vi "Main.vi"() -> ()   [LabVIEW 2014]
doc: "This Continuous Measurement sample project is based on the Queued Message Handler template.\n\nThe Event Handling Loop generates messages based on user interface actions.\n\nThe Message Handling Loop processes messages generated by the Event Handling Loop, or by other messages. There are also Acquisition and Logging message handling loop subVIs, and a chart updating loop."
uses:
  eod2016/controls/Recording Metadata.ctl
  Settings/Settings.ctl
  Acquisition/Hardware Configuration.ctl
  Logging/Logging Configuration.ctl
  controls/UI Data.ctl
  controls/UI State.ctl
  support/Message Queue/Enqueue Message (Single).vi
  <vilib>/Utility/error.llb/Error Cluster From Error Code.vi
  <vilib>/ErrorRing/Error Ring.xnode
  Acquisition/Acquisition.lvlib
  Logging/Logging.lvlib
  Settings/Settings.lvlib
  support/User Event - Stop/User Event - Stop.lvlib
  support/Message Queue/Message Queue.lvlib
panel:
  in  "UserMetaData":T1 {"Amplifier Model" items=["Select a Model", "AM 1700", "BMA 200"]}
  out "Data":waveform(dbl)[](graph)
  in  "Settings":bool
  in  "Start":bool
  in  "Stop":bool
  out "Status":string
  in  "Exit":bool
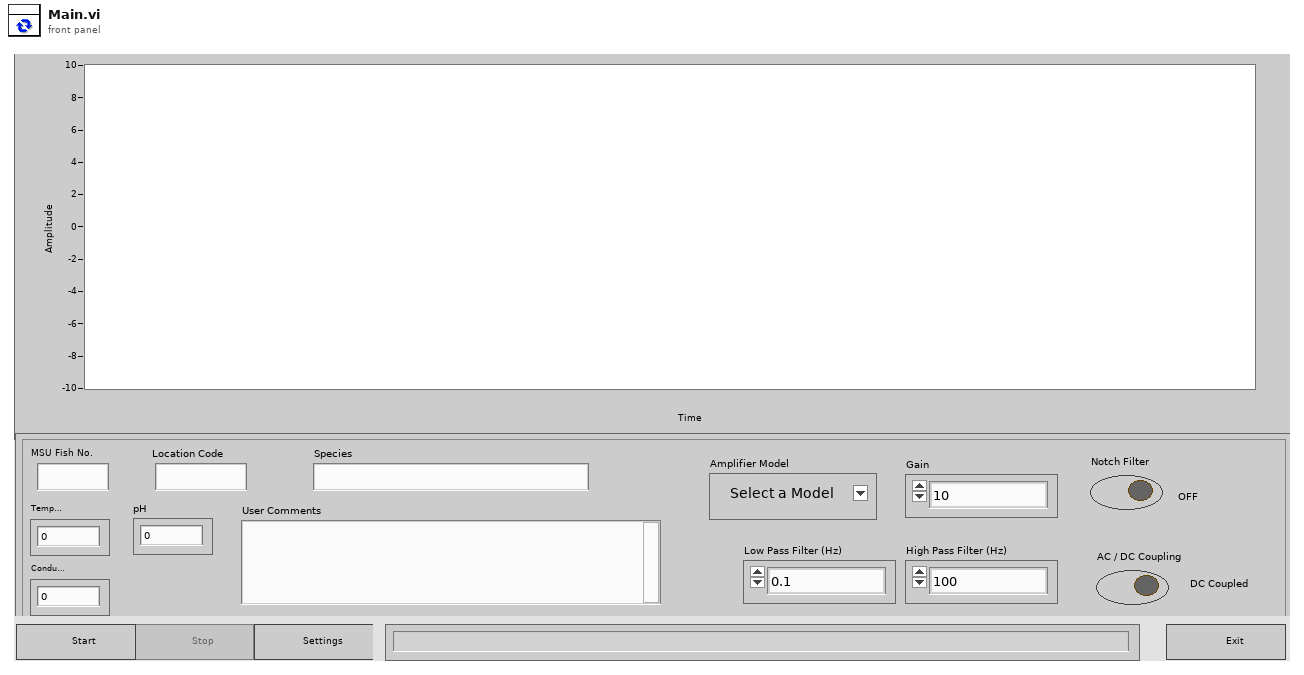
[diagram p1: front panel]
types:
  T1 = typedef "Recording Metadata.ctl" = cluster{"MSU Fish No.":string, "Location Code":string, "Species":string, "Temperature":dbl, "pH":dbl, "Conductivity":dbl, "User Comments":string, "Amplifier Model":u16, "Gain":enum16{"10", "20", "50", "100", "200", "500", "1000", "2k", "5k", "10k", "20k", "50k"}, "Low Pass Filter (Hz)":enum16{"0.1", "1", "3", "10", "30", "100", "300"}, "High Pass Filter (Hz)":enum16{"100", "500", "1000", "3000", "5000", "10,000", "20,000", "30,000", "50,000"}, "AC / DC Coupling":bool, "Notch Filter":bool}
  T2 = typedef "UI State.ctl" = enum16{"Idle", "Acquiring and Logging", "Waiting for Exit", "Waiting for Exit (Acq Stopped)", "Waiting for Exit (Log Stopped)", "Waiting for Stop", "Waiting for Stop (Acq Stopped)", "Waiting for Stop (Log Stopped)"}
  T3 = typedef "UI Data.ctl" = cluster{"Start Ref":refnum<vi>, "Trigger Ref":refnum<vi>, "Stop Ref":refnum<vi>, "Settings Ref":refnum<vi>, "Status Ref":refnum<vi>, "Exit Ref":refnum<vi>, "Data Ref":refnum<vi>}
  T4 = typedef "Settings.lvlib/Settings.ctl" = cluster{"Hardware Configuration":T5, "Logging Configuration":T6}
  T5 = typedef "Acquisition.lvlib/Hardware Configuration.ctl" = cluster{"DAQmx Channel":tag, "Max Input":dbl, "Min Input":dbl, "Sample Rate":dbl, "DAQmx Task":refnum<k21>}
  T6 = typedef "Logging.lvlib/Logging Configuration.ctl" = cluster{"Log File Base Path":path, "TDMS File Reference":refnum<k34>, "Samples to Save":u32, "InterRecording Delay":dbl}
  T7 = typedef "Message Queue.lvlib/All Message Queues.ctl" = cluster{"UI":refnum<queue>, "Acquisition":refnum<queue>, "Logging":refnum<queue>, "Timer":refnum<queue>}
  T8 = enum8{"Enabled", "Disabled", "Disabled and Grayed Out"}
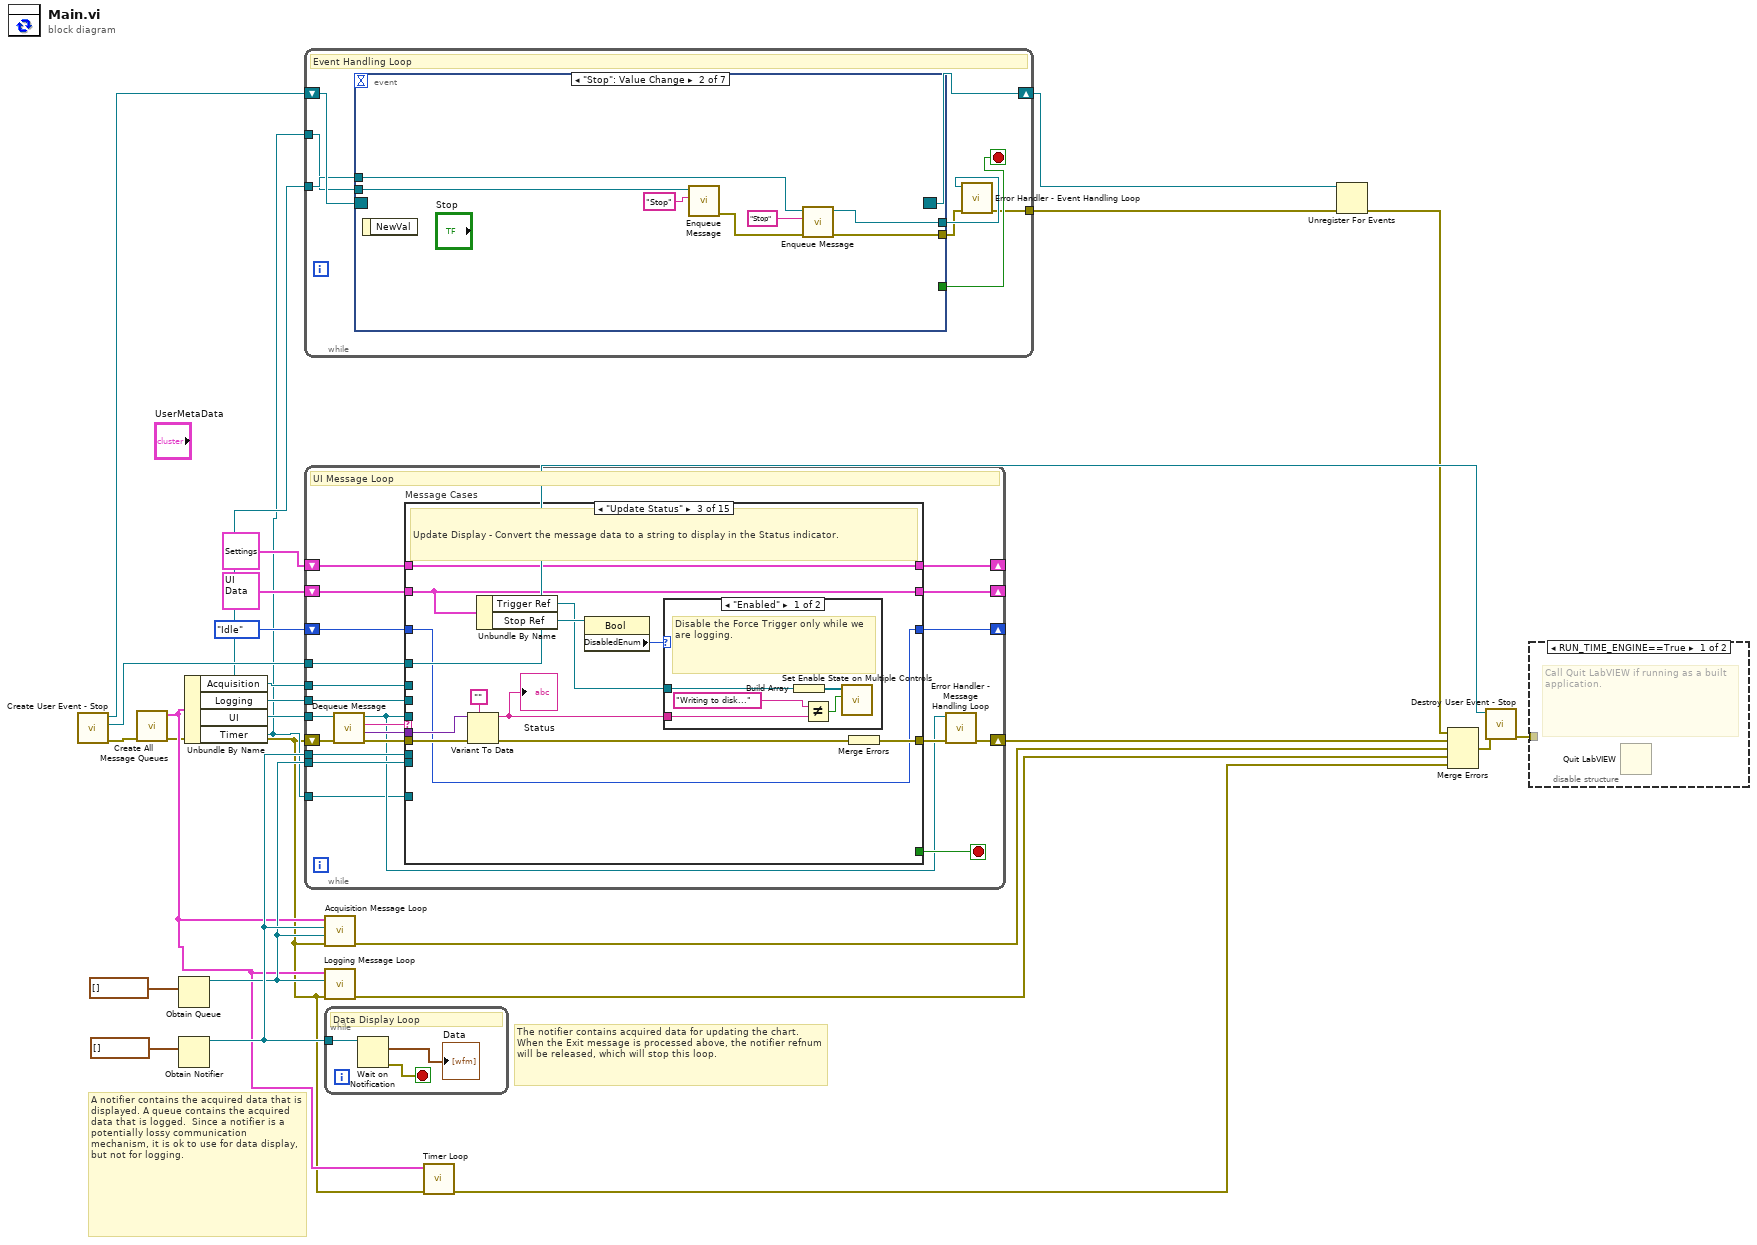
[diagram p0: block diagram]
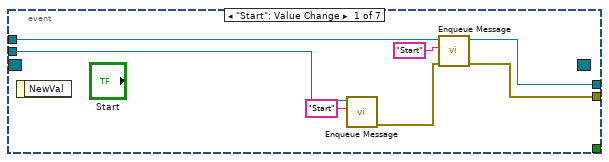
[diagram p3: hidden frame]
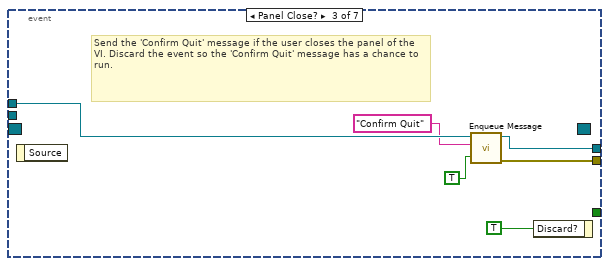
[diagram p4: hidden frame]
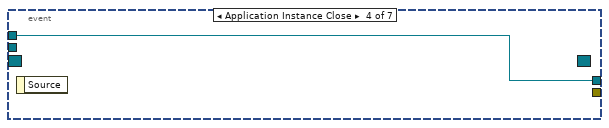
[diagram p5: hidden frame]
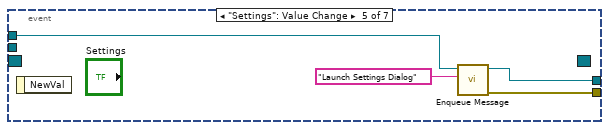
[diagram p6: hidden frame]
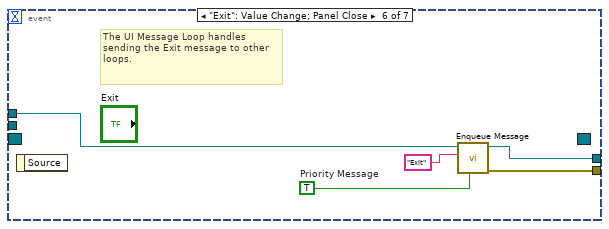
[diagram p7: hidden frame]
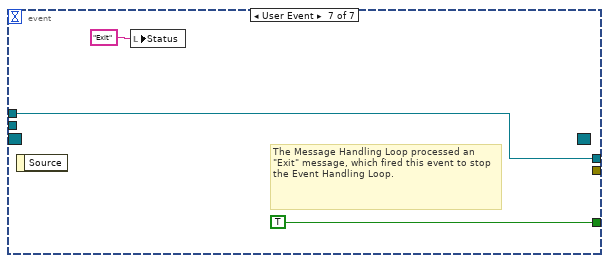
[diagram p8: hidden frame]
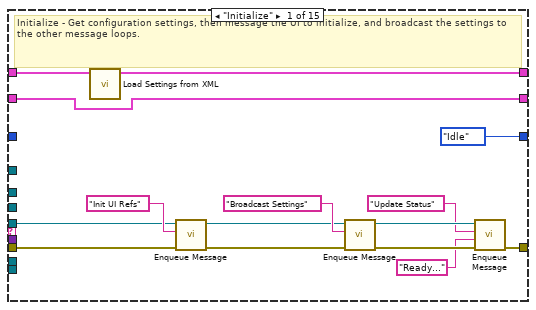
[diagram p9: hidden frame]
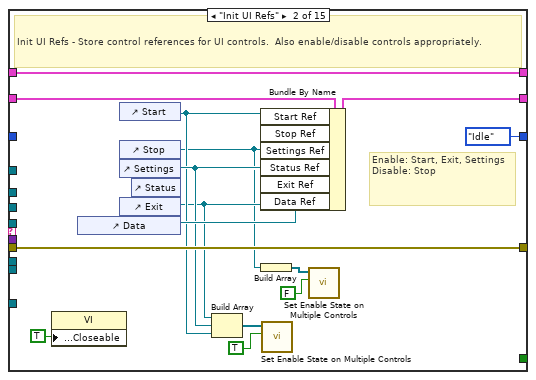
[diagram p10: hidden frame]
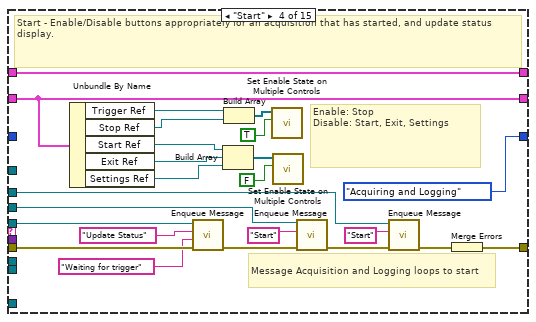
[diagram p12: hidden frame]
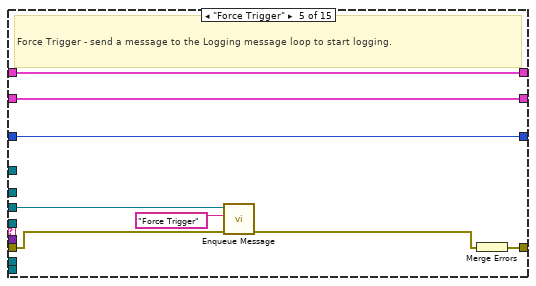
[diagram p13: hidden frame]
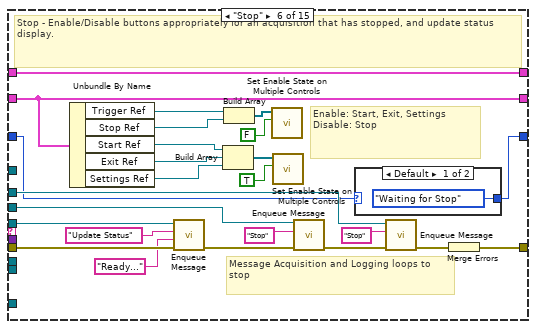
[diagram p14: hidden frame]
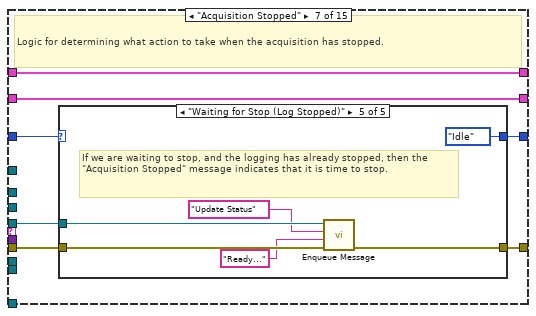
[diagram p16: hidden frame]
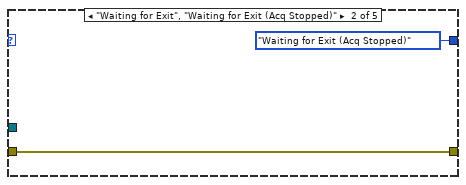
[diagram p18: hidden frame]
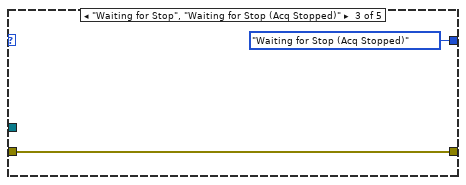
[diagram p19: hidden frame]
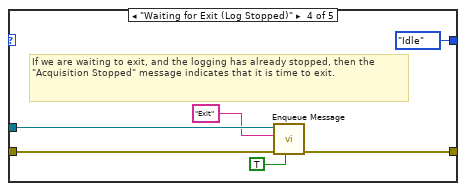
[diagram p20: hidden frame]
diagram:
  # "A notifier contains the acquired data that is displayed. A queue contains the acquired data that is logged.  Since a notifier is a potentially lossy communication mechanism, it is ok to use for data display, but not for logging."
  # "The notifier contains acquired data for updating the chart. When the Exit message is processed above, the notifier refnum will be released, which will stop this loop."
  n1 = call "Create User Event - Stop.vi"() -> ("error out"=w19:errorcluster, "User Event - Stop"=w21:refnum<user-event>, "Stop Event Registration Refnum"=w22:refnum<event-registration>)  [unwired: 9 in]
  n2 = call "Create All Message Queues.vi"("error in (no error)"=w19) -> ("error out"=w2:errorcluster, "Message Queues out"=w3:T7)  [unwired: 9 in]
  n3 = Obtain Queue(element data type=waveform(dbl)[] []) -> (queue out=w9:refnum<queue>)  [unwired: 4 in, 2 out]
  n4 = Obtain Notifier(notification data type=waveform(dbl)[] []) -> (notifier out=w11:refnum<notifier>)  [unwired: 3 in, 2 out]
  n5 = Unbundle By Name(w3) -> ("Acquisition"=w14:refnum<queue>, "Logging"=w13:refnum<queue>, "UI"=w6:refnum<queue>, "Timer"=w4:refnum<queue>)
  n6 = while {
    tunnel: w6 -> [w32]
    tunnel: [w27] -> w24
    shift-right: [w31] -> w16
    shift-left: w22 -> [w33]
    tunnel: w4 -> [w26]
    stop <- w30 stop-if-true
    # "Event Handling Loop"
    n7 = event shown="[1] \"Stop\": Value Change" {
      selector: w33 -> [_ _ _ _ _ _ _]
      dyn-events: [_ _ _ _ _ _ _] -> w31
      timeout: _ -> [_ _ _ _ _ _ _]
      tunnel: [_ _ _ _ _ _ TRUE ("Discard?")] -> w30
      tunnel: w32 -> [w38 w46 w53 w54 w56 w60 w64]
      tunnel: [w40 w45 w48 _ w58 w63 _] -> w28
      tunnel: [w37 w44 w49 w54 w55 w59 w64] -> w29
      tunnel: w26 -> [w35 w43 _ _ _ _ _]
      event "Start": Value Change {
        n8 = event-data() -> ()  [unwired: 1 in, 1 out]
        n9 = call-poly "Enqueue Message.vi"("Message"="Start", "Message Queue"=w35) -> ("error out"=w36:errorcluster)  [unwired: 8 in, 1 out]
        n10 = call-poly "Enqueue Message.vi"("error in (no error)"=w36, "Message"="Start", "Message Queue"=w38) -> ("error out"=w40:errorcluster, "dup Message Queue"=w37:refnum<queue>)  [unwired: 7 in]
      }
      event "Stop": Value Change {
        n11 = event-data() -> ()  [unwired: 1 in, 1 out]
        n12 = call-poly "Enqueue Message.vi"("Message"="Stop", "Message Queue"=w43) -> ("error out"=w42:errorcluster)  [unwired: 8 in, 1 out]
        n13 = call-poly "Enqueue Message.vi"("error in (no error)"=w42, "Message"="Stop", "Message Queue"=w46) -> ("error out"=w45:errorcluster, "dup Message Queue"=w44:refnum<queue>)  [unwired: 7 in]
      }
      event Panel Close? {
        # "Send the 'Confirm Quit' message if the user closes the panel of the VI. Discard the event so the 'Confirm Quit' message has a chance to run."
        n14 = event-data() -> ()  [unwired: 1 in, 1 out]
        n15 = call-poly "Enqueue Message.vi"("Priority Message? (F)"=TRUE, "Message"="Confirm Quit", "Message Queue"=w53) -> ("error out"=w48:errorcluster, "dup Message Queue"=w49:refnum<queue>)  [unwired: 7 in]
        n16 = event-data("Discard?"=TRUE) -> ()  [unwired: 1 in, 1 out]
      }
      event Application Instance Close {
        n17 = event-data() -> ()  [unwired: 1 in, 1 out]
      }
      event "Settings": Value Change {
        n18 = event-data() -> ()  [unwired: 1 in, 1 out]
        n19 = call-poly "Enqueue Message.vi"("Message"="Launch Settings Dialog", "Message Queue"=w56) -> ("error out"=w58:errorcluster, "dup Message Queue"=w55:refnum<queue>)  [unwired: 8 in]
      }
      event "Exit": Value Change; Panel Close {
        w61 = TRUE  # Priority Message
        # "The UI Message Loop handles sending the Exit message to other loops."
        n20 = event-data() -> ()  [unwired: 1 in, 1 out]
        n21 = call-poly "Enqueue Message.vi"("Priority Message? (F)"=w61, "Message"="Exit", "Message Queue"=w60) -> ("error out"=w63:errorcluster, "dup Message Queue"=w59:refnum<queue>)  [unwired: 7 in]
      }
      event User Event {
        # "The Message Handling Loop processed an \"Exit\" message, which fired this event to stop the Event Handling Loop."
        n22 = event-data() -> ()  [unwired: 1 in, 1 out]
        n23 = local write "Status"("Exit" ("Exit String")) -> ()
      }
    }
    n24 = call "Error Handler - Event Handling Loop.vi"("error in (no error)"=w28, "Message Queue"=w29) -> ("dup error in"=w27:errorcluster)  [unwired: 8 in, 1 out]
  }
  n25 = while {
    tunnel: w6 -> [w81]
    tunnel: w21 -> [w86]
    shift-right: [w71] -> w25
    shift-left: w2 -> [w85]
    shift-right: [w80] -> _
    shift-left: T4 {"Hardware Configuration"={"DAQmx Channel"="", "Max Input"=0.0, "Min Input"=0.0, "Sample Rate"=0.0, "DAQmx Task"=""}, "Logging Configuration"={"Log File Base Path"=path "", "TDMS File Reference"=refnum, "Samples to Save"=0, "InterRecording Delay"=0.0}} ("Settings") -> [w79]
    shift-right: [w77] -> _
    shift-left: T3 {"Start Ref"=refnum, "Trigger Ref"=refnum, "Stop Ref"=refnum, "Settings Ref"=refnum, "Status Ref"=refnum, "Exit Ref"=refnum, "Data Ref"=refnum} ("Measurement UI Controls") -> [w78]
    tunnel: w14 -> [w76]
    tunnel: w13 -> [w75]
    tunnel: w11 -> [w74]
    tunnel: w9 -> [w73]
    shift-right: [w68] -> _
    shift-left: UI_State."Idle" ("UI State") -> [w69]
    tunnel: w4 -> [w67]
    stop <- w87 stop-if-true
    # "UI Message Loop"
    n26 = call "Dequeue Message.vi"("error in (no error)"=w85, "Message Queue"=w81) -> ("error out"=w84:errorcluster, "Message Data"=w82:variant, "Message"=w83:string, "dup Message Queue"=w70:refnum<queue>)  [unwired: 6 in]
    n27 = case "Message Cases" shown="\"Update Status\"" w83 {
      selector: w83 -> [_ _ _ _ _ _ _ _ _ _ _ _ _ _ w339]
      tunnel: w70 -> [w92 _ _ w158 _ w191 w195 w220 _ w264 w279 w289 w322 _ _]
      tunnel: w84 -> [w91 w118 w129 w157 w164 w190 w197 w222 w254 w266 w283 w288 w330 w337 _]
      tunnel: [w98 w118 w130 w159 w167 w192 w196 w221 w258 w261 w274 w287 w331 w336 w340] -> w72
      tunnel: [_ _ _ _ _ _ _ _ _ _ _ _ TRUE _ _] -> w87
      tunnel: w82 -> [_ _ w128 _ _ _ _ _ _ _ w282 _ _ _ _]
      tunnel: w86 -> [_ _ _ _ _ _ _ _ _ _ _ _ w329 _ _]
      tunnel: [w101 w117 w125 w156 w166 w189 w201 w226 w256 w263 w285 w292 w327 w335 w342] -> w80
      tunnel: w79 -> [w102 w117 w125 w156 w166 w189 w201 w226 w256 w267 w285 w292 w327 w335 w342]
      tunnel: w78 -> [w94 w116 w124 w153 w165 w186 w200 w225 w253 w260 w284 w291 w325 w334 w341]
      tunnel: [w94 w115 w124 w153 w165 w186 w200 w225 w253 w260 w284 w291 w325 w334 w341] -> w77
      tunnel: w76 -> [_ _ _ w140 _ w173 _ _ w252 _ _ _ w324 _ _]
      tunnel: w75 -> [_ _ _ w143 w161 w176 _ _ w251 _ _ _ w323 _ _]
      tunnel: w74 -> [_ _ _ _ _ _ _ _ _ _ _ _ w321 _ _]
      tunnel: w73 -> [_ _ _ _ _ _ _ _ _ _ _ _ w317 _ _]
      tunnel: w69 -> [_ _ w119 _ w160 w169 w199 w224 w250 w259 w273 w290 _ w333 w338]
      tunnel: [UI_State."Idle" ("UI State") UI_State."Idle" ("UI State") w119 UI_State."Acquiring and Logging" ("UI State") w160 w168 w198 w223 w250 w259 w273 w286 UI_State."Idle" ("UI State") w333 w338] -> w68
      tunnel: w67 -> [_ _ _ _ _ _ _ _ w249 _ _ _ _ _ _]
      frame "Initialize" {
        # "Initialize - Get configuration settings, then message the UI to initialize, and broadcast the settings to the other message loops."
        n28 = call "Load Settings from XML.vi"("Settings in"=w102) -> ("Settings out"=w101:T4)  [unwired: 9 in, 1 out]
        n29 = call-poly "Enqueue Message.vi"("error in (no error)"=w91, "Message"="Init UI Refs", "Message Queue"=w92) -> ("error out"=w89:errorcluster, "dup Message Queue"=w90:refnum<queue>)  [unwired: 7 in]
        n30 = call-poly "Enqueue Message.vi"("error in (no error)"=w89, "Message"="Broadcast Settings", "Message Queue"=w90) -> ("error out"=w100:errorcluster, "dup Message Queue"=w99:refnum<queue>)  [unwired: 7 in]
        n31 = call-poly "Enqueue Message.vi"("error in (no error)"=w100, "Message Data"="Ready..." ("Ready..."), "Message"="Update Status", "Message Queue"=w99) -> ("error out"=w98:errorcluster)  [unwired: 6 in, 1 out]
      }
      frame "Init UI Refs" {
        # "Enable: Start, Exit, Settings\nDisable: Stop"
        # "Init UI Refs - Store control references for UI controls.  Also enable/disable controls appropriately."
        n32 = property class="VI"("Front Panel.Closeable"=TRUE ("Front Panel Window:Closeable")) -> ()  [unwired: 2 in, 2 out]
        n33 = control-ref of="Data"() -> (w111:refnum<vi>)
        n34 = control-ref of="Start"() -> (w110:refnum<vi>)
        n35 = control-ref of="Stop"() -> (w105:refnum<vi>)
        n36 = control-ref of="Settings"() -> (w107:refnum<vi>)
        n37 = control-ref of="Exit"() -> (w106:refnum<vi>)
        n38 = control-ref of="Status"() -> (w112:refnum<vi>)
        n39 = Build Array(w106, w107, w110) -> (w109:refnum<vi>[])
        n40 = Bundle By Name(cluster=w116, "Start Ref"=w110, "Stop Ref"=w105, "Settings Ref"=w107, "Status Ref"=w112, "Exit Ref"=w106, "Data Ref"=w111) -> (w115:T3)
        n41 = Build Array(w105) -> (w104:refnum<vi>[])
        n42 = call "Set Enable State on Multiple Controls.vi"("Enable?"=TRUE, "Controls"=w109) -> ()  [unwired: 10 in]
        n43 = call "Set Enable State on Multiple Controls.vi"("Enable?"=FALSE, "Controls"=w104) -> ()  [unwired: 10 in]
      }
      frame "Update Status" {
        # "Update Display - Convert the message data to a string to display in the Status indicator."
        n44 = Variant To Data(error in=w129, type="", Variant=w128) -> (data=w121:string, error out=w126:errorcluster)
        "Status" <- w121
        n45 = Unbundle By Name(w124) -> ("Trigger Ref"=w120:refnum<vi>, "Stop Ref"=w123:refnum<vi>)
        n46 = property class="Bool"(reference=w123) -> ("DisabledEnum"=w122:T8)  [unwired: 1 in, 2 out]
        n47 = case shown="\"Enabled\"" w122 {
          tunnel: w121 -> [w133 _]
          tunnel: w120 -> [w134 _]
          frame "Enabled" {
            # "Disable the Force Trigger only while we are logging."
            n48 = Build Array(w134) -> (w135:refnum<vi>[])
            n49 = Not Equal?(x="Writing to disk..." ("Logging"), y=w133) -> (x != y?=w131:bool)
            n50 = call "Set Enable State on Multiple Controls.vi"("Enable?"=w131, "Controls"=w135) -> ()  [unwired: 10 in]
          }
          frame "Disabled", Default {
          }
        }
        n51 = Merge Errors(w126) -> (w130:errorcluster)
      }
      frame "Start" {
        # "Message Acquisition and Logging loops to start"
        # "Enable: Stop\nDisable: Start, Exit, Settings"
        # "Start - Enable/Disable buttons appropriately for an acquisition that has started, and update status display."
        n52 = Unbundle By Name(w153) -> ("Trigger Ref"=w137:refnum<vi>, "Stop Ref"=w138:refnum<vi>, "Start Ref"=w148:refnum<vi>, "Exit Ref"=w147:refnum<vi>, "Settings Ref"=w146:refnum<vi>)
        n53 = call-poly "Enqueue Message.vi"("error in (no error)"=w157, "Message Data"="Waiting for trigger" ("Waiting for trigger"), "Message"="Update Status", "Message Queue"=w158) -> ("error out"=w145:errorcluster)  [unwired: 6 in, 1 out]
        n54 = Build Array(w148, w147, w146) -> (w151:refnum<vi>[])
        n55 = Build Array(w137, w138) -> (w150:refnum<vi>[])
        n56 = call "Set Enable State on Multiple Controls.vi"("Enable?"=TRUE, "Controls"=w150) -> ()  [unwired: 10 in]
        n57 = call "Set Enable State on Multiple Controls.vi"("Enable?"=FALSE, "Controls"=w151) -> ()  [unwired: 10 in]
        n58 = call-poly "Enqueue Message.vi"("error in (no error)"=w145, "Message"="Start", "Message Queue"=w143) -> ("error out"=w142:errorcluster)  [unwired: 7 in, 1 out]
        n59 = call-poly "Enqueue Message.vi"("error in (no error)"=w142, "Message"="Start", "Message Queue"=w140) -> ("error out"=w141:errorcluster)  [unwired: 7 in, 1 out]
        n60 = Merge Errors(w141) -> (w159:errorcluster)
      }
      frame "Force Trigger" {
        # "Force Trigger - send a message to the Logging message loop to start logging."
        n61 = call-poly "Enqueue Message.vi"("error in (no error)"=w164, "Message"="Force Trigger", "Message Queue"=w161) -> ("error out"=w163:errorcluster)  [unwired: 7 in, 1 out]
        n62 = Merge Errors(w163) -> (w167:errorcluster)
      }
      frame "Stop" {
        # "Message Acquisition and Logging loops to stop"
        # "Enable: Start, Exit, Settings\nDisable: Stop"
        # "Stop - Enable/Disable buttons appropriately for an acquisition that has stopped, and update status display."
        n63 = Unbundle By Name(w186) -> ("Trigger Ref"=w170:refnum<vi>, "Stop Ref"=w171:refnum<vi>, "Start Ref"=w181:refnum<vi>, "Exit Ref"=w180:refnum<vi>, "Settings Ref"=w179:refnum<vi>)
        n64 = call-poly "Enqueue Message.vi"("error in (no error)"=w190, "Message Data"="Ready..." ("Ready..."), "Message"="Update Status", "Message Queue"=w191) -> ("error out"=w178:errorcluster)  [unwired: 6 in, 1 out]
        n65 = Build Array(w181, w180, w179) -> (w184:refnum<vi>[])
        n66 = Build Array(w170, w171) -> (w183:refnum<vi>[])
        n67 = call "Set Enable State on Multiple Controls.vi"("Enable?"=FALSE, "Controls"=w183) -> ()  [unwired: 10 in]
        n68 = call "Set Enable State on Multiple Controls.vi"("Enable?"=TRUE, "Controls"=w184) -> ()  [unwired: 10 in]
        n69 = call-poly "Enqueue Message.vi"("error in (no error)"=w178, "Message"="Stop", "Message Queue"=w176) -> ("error out"=w175:errorcluster)  [unwired: 7 in, 1 out]
        n70 = case shown="Default" w169 {
          selector: w169 -> [_ w194]
          tunnel: [UI_State."Waiting for Stop" ("UI State") w194] -> w168
          frame Default {
          }
          frame "Waiting for Exit" {
          }
        }
        n71 = call-poly "Enqueue Message.vi"("error in (no error)"=w175, "Message"="Stop", "Message Queue"=w173) -> ("error out"=w174:errorcluster)  [unwired: 7 in, 1 out]
        n72 = Merge Errors(w174) -> (w192:errorcluster)
      }
      frame "Acquisition Stopped" {
        # "Logic for determining what action to take when the acquisition has stopped."
        n73 = case shown="\"Waiting for Stop (Log Stopped)\"" w199 {
          selector: w199 -> [w203 _ _ _ _]
          tunnel: [w203 UI_State."Waiting for Exit (Acq Stopped)" ("UI State") UI_State."Waiting for Stop (Acq Stopped)" ("UI State") UI_State."Idle" ("UI State") UI_State."Idle" ("UI State")] -> w198
          tunnel: w197 -> [w202 w204 w206 w212 w218]
          tunnel: [w202 w204 w206 w211 w217] -> w196
          tunnel: w195 -> [_ _ _ w210 w216]
          frame Default {
          }
          frame "Waiting for Exit", "Waiting for Exit (Acq Stopped)" {
          }
          frame "Waiting for Stop", "Waiting for Stop (Acq Stopped)" {
          }
          frame "Waiting for Exit (Log Stopped)" {
            # "If we are waiting to exit, and the logging has already stopped, then the \"Acquisition Stopped\" message indicates that it is time to exit."
            n74 = call-poly "Enqueue Message.vi"("Priority Message? (F)"=TRUE, "error in (no error)"=w212, "Message"="Exit", "Message Queue"=w210) -> ("error out"=w211:errorcluster)  [unwired: 6 in, 1 out]
          }
          frame "Waiting for Stop (Log Stopped)" {
            # "If we are waiting to stop, and the logging has already stopped, then the \"Acquisition Stopped\" message indicates that it is time to stop."
            n75 = call-poly "Enqueue Message.vi"("error in (no error)"=w218, "Message Data"="Ready..." ("Message"), "Message"="Update Status", "Message Queue"=w216) -> ("error out"=w217:errorcluster)  [unwired: 6 in, 1 out]
          }
        }
      }
      frame "Logging Stopped" {
        # "Logic for determining what action to take when the logging has stopped."
        n76 = case shown="\"Waiting for Stop (Acq Stopped)\"" w224 {
          selector: w224 -> [w228 _ _ _ _]
          tunnel: [w228 UI_State."Waiting for Exit (Log Stopped)" ("UI State") UI_State."Waiting for Stop (Log Stopped)" ("UI State") UI_State."Idle" ("UI State") UI_State."Idle" ("UI State")] -> w223
          tunnel: w222 -> [w227 w229 w231 w237 w243]
          tunnel: [w227 w229 w231 w236 w242] -> w221
          tunnel: w220 -> [_ _ _ w235 w241]
          frame Default {
          }
          frame "Waiting for Exit", "Waiting for Exit (Log Stopped)" {
          }
          frame "Waiting for Stop", "Waiting for Stop (Log Stopped)" {
          }
          frame "Waiting for Exit (Acq Stopped)" {
            # "If we are waiting to exit, and the acquisition has already stopped, then the \"Logging Stopped\" message indicates that it is time to exit."
            n77 = call-poly "Enqueue Message.vi"("Priority Message? (F)"=TRUE, "error in (no error)"=w237, "Message"="Exit", "Message Queue"=w235) -> ("error out"=w236:errorcluster)  [unwired: 6 in, 1 out]
          }
          frame "Waiting for Stop (Acq Stopped)" {
            # "If we are waiting to stop, and the acquisition has already stopped, then the \"Logging Stopped\" message indicates that it is time to stop."
            n78 = call-poly "Enqueue Message.vi"("error in (no error)"=w243, "Message Data"="Ready..." ("Message"), "Message"="Update Status", "Message Queue"=w241) -> ("error out"=w242:errorcluster)  [unwired: 6 in, 1 out]
          }
        }
      }
      frame "Broadcast settings" {
        w246 = "Update Settings" ("Message")
        # "Send the 'Update Settings' message to the Logging and Acquisition message loops."
        n79 = Unbundle By Name(w256) -> ("Hardware Configuration"=w255:T5, "Logging Configuration"=w245:T6)
        n80 = call-poly "Enqueue Message.vi"("Message Data"=w255, "Message"=w246, "Message Queue"=w252) -> ("error out"=w257:errorcluster)  [unwired: 7 in, 1 out]
        n81 = call-poly "Enqueue Message.vi"("error in (no error)"=w257, "Message Data"=w245, "Message"=w246, "Message Queue"=w251) -> ("error out"=w248:errorcluster)  [unwired: 6 in, 1 out]
        n82 = call-poly "Enqueue Message.vi"("error in (no error)"=w248, "Message Data"=w245, "Message"=w246, "Message Queue"=w249) -> ("error out"=w247:errorcluster)  [unwired: 6 in, 1 out]
        n83 = Merge Errors(w247, w254) -> (w258:errorcluster)
      }
      frame "Launch Settings Dialog" {
        # "Launch the Settings Dialog when the user clicks the 'Settings' button."
        n84 = call "Settings Dialog.vi"("error in (no error)"=w266, "Settings in"=w267) -> ("error out"=w262:errorcluster, "Cancelled?"=w265:bool, "Settings out"=w263:T4)  [unwired: 6 in, 1 out]
        n85 = case shown="False" w265 {
          tunnel: w264 -> [w271 _]
          tunnel: w262 -> [w270 w272]
          tunnel: [w269 w272] -> w261
          frame False {
            n86 = call-poly "Enqueue Message.vi"("error in (no error)"=w270, "Message"="Broadcast Settings", "Message Queue"=w271) -> ("error out"=w269:errorcluster)  [unwired: 7 in, 1 out]
          }
          frame True {
          }
        }
      }
      frame "Error" {
        # "Error - Check the error message data and respond accordingly. This message is sent by the \"Error Handler\" VIs at the end of each loop in this application."
        n87 = Variant To Data(error in=w283, type=errorcluster {"status"=FALSE, "code"=0, "source"=""} ("error out"), Variant=w282) -> (data=w280:errorcluster, error out=w276:errorcluster)
        n88 = call <vilib>:"Simple Error Handler.vi"("error in (no error)"=w280) -> ()  [unwired: 4 in, 5 out]
        n89 = call-poly "Enqueue Message.vi"("Priority Message? (F)"=TRUE, "Message"="Exit", "Message Queue"=w279) -> ("error out"=w275:errorcluster)  [unwired: 7 in, 1 out]
        n90 = Merge Errors(w275, w276) -> (w274:errorcluster)
      }
      frame "Confirm Quit" {
        # "Confirm Quit - Message that can confirm whether or not the user wants to exit the application."
        n91 = case shown="\"Acquiring and Logging\"" w290 {
          tunnel: w289 -> [w297 w303]
          tunnel: w288 -> [w296 w301]
          tunnel: [w293 w300] -> w287
          tunnel: [UI_State."Idle" ("UI State") w299] -> w286
          frame Default {
            # "If 'Confirm Quit' comes in while the system is idle, there is no need for a confirmation message."
            n92 = call-poly "Enqueue Message.vi"("Priority Message? (F)"=TRUE, "error in (no error)"=w296, "Message"="Exit", "Message Queue"=w297) -> ("error out"=w293:errorcluster)  [unwired: 6 in, 1 out]
          }
          frame "Acquiring and Logging" {
            n93 = Two Button Dialog(message="Are you sure you want to quit while the acquisition is running?" ("Confirm Quit Message"), 1:"No" ("No"), 2:"Yes" ("Yes")) -> (T button?=w302:bool)
            n94 = case shown="True" w302 {
              tunnel: w303 -> [_ w313]
              tunnel: w301 -> [w307 w312]
              tunnel: [w307 w311] -> w300
              tunnel: [UI_State."Acquiring and Logging" ("UI State") UI_State."Waiting for Exit" ("UI State")] -> w299
              frame False {
                # "User did not want to quit."
              }
              frame True {
                n95 = call-poly "Enqueue Message.vi"("error in (no error)"=w312, "Message"="Stop", "Message Queue"=w313) -> ("error out"=w311:errorcluster)  [unwired: 7 in, 1 out]
              }
            }
          }
        }
      }
      frame "Exit" {
        w326 = "Exit" ("Message")
        # "Don't check the error outs. The acquisition and logging queues may have already been released."
        # "Close references owned by the Main VI."
        # "Stop the VI"
        # "Exit - Fire the User Event to stop the Event Handling Loop.  Also send Exit messages to the Acquisition and Logging loops."
        n96 = Release Queue(queue=w322, error in (no error)=w330) -> (error out=w320:errorcluster)  [unwired: 1 in, 2 out]
        n97 = call "Fire User Event - Stop.vi"("User Event - Stop"=w329) -> ("error out"=w328:errorcluster)  [unwired: 10 in]
        n98 = Release Notifier(notifier=w321, error in (no error)=w320) -> (error out=w319:errorcluster)  [unwired: 1 in, 2 out]
        n99 = Release Queue(queue=w317, error in (no error)=w319) -> (error out=w318:errorcluster)  [unwired: 1 in, 2 out]
        n100 = call-poly "Enqueue Message.vi"("Priority Message? (F)"=TRUE, "Message"=w326, "Message Queue"=w324) -> ()  [unwired: 7 in, 2 out]
        n101 = call-poly "Enqueue Message.vi"("Priority Message? (F)"=TRUE, "Message"=w326, "Message Queue"=w323) -> ()  [unwired: 7 in, 2 out]
        n102 = Merge Errors(w328, w318) -> (w331:errorcluster)
      }
      frame "---Copy This Frame---" {
        # "Duplicate this frame when creating new messages.  Change this comment in the duplicated frame to describe this message."
        n103 = Merge Errors(w337) -> (w336:errorcluster)
      }
      frame Default {
        # "'Default' case only runs if there is a message that isn't defined in any of the other cases.  Output a programming error."
        n104 = xnode "Error Ring"("parameter 0"=w339) -> ("error out"=w340:errorcluster)
      }
    }
    n105 = call "Error Handler - Message Handling Loop.vi"("error in (no error)"=w72, "Message Queue"=w70) -> ("dup error in"=w71:errorcluster)  [unwired: 8 in, 1 out]
  }
  n106 = call "Acquisition Message Loop.vi"("error in (no error)"=w2, "Data Queue"=w9, "Data Notifier"=w11, "Message Queues"=w3) -> ("error out"=w20:errorcluster)  [unwired: 7 in]
  n107 = call "Logging Message Loop.vi"("error in (no error)"=w2, "Data Queue"=w9, "Message Queues"=w3) -> ("error out"=w18:errorcluster)  [unwired: 8 in]
  n108 = while "Data Display Loop" {
    tunnel: w11 -> [w352]
    stop <- w350 stop-if-true
    # "Data Display Loop"
    n109 = Wait on Notification(notifier=w352) -> (notification=→"Data":waveform(dbl)[], error out=w350:errorcluster)  [unwired: 3 in, 2 out]
  }
  n110 = call "Timer Loop.vi"("error in (no error)"=w2, "Message Queues"=w3) -> ("error out"=w1:errorcluster)  [unwired: 9 in]
  n111 = Unregister For Events(event registration refnum=w16, error in=w24) -> (error out=w17:errorcluster)
  n112 = Merge Errors(w17, w25, w20, w18, w1) -> (w23:errorcluster)
  n113 = call "Destroy User Event - Stop.vi"("error in (no error)"=w23, "User Event - Stop"=w21) -> ("error out"=w8:errorcluster)  [unwired: 9 in]
  n114 = disable-structure shown="RUN_TIME_ENGINE==True" {
    disable-tunnel: w8 -> [_ _]
    frame condition #0 {
      # "Call Quit LabVIEW if running as a built application."
      n115 = Quit LabVIEW() -> ()  [unwired: 1 in]
    }
    frame condition #1 (active) {
    }
  }
